vi "read_dust_control_settings_big.vi"(7 "Settings to be loaded":i32=-1, 8 "error in (no error)":errorcluster, 9 "Query Cluster":T1, 10 "Lower Timestamp Range":timestamp, 11 "Upper Timestamp Range":timestamp) -> (0 "error out":errorcluster, 1 "Settings Array":cluster{"String":string, "Value":dbl}[](array[cluster]), 3 "Dust Source Array":T2[](array[typedef]) {"Needle Voltage" min=0.0 max=10.0 step=0.01 format="%.2g"; "Y Voltage" min=0.0 max=9.0 step=0.01 format="%.2g"; "X Voltage" min=0.0 max=9.0 step=0.01 format="%.2g"; "Einzel Voltage" min=0.0 max=10.0 step=0.01 format="%.2g"; "Desired Amplitude (V)" min=0.0 max=10.0 step=0.01 format="%5.2f"; "Width (ms) : 0.1" min=0.05 max=5.0 step=0.01 format="%6.2f"; "Frequency" min=1.0 max=100.0 step=0.01 format="%.1f"})   [LabVIEW 2013]
doc: "Returns an array of events from the source_settings table based on the tag, dust type, high voltage, and id_source_settings, if specified. Unless a specific id_source_settings is requested, an uppper timestamp range and lower timestamp range are necessary."
uses:
  User Interface/Controls/dust_source_control.ctl
  <vilib>/addons/database/_DB Variant To Data/Database Variant To Data.xnode
panel:
  out "SQL Query Syntax":string
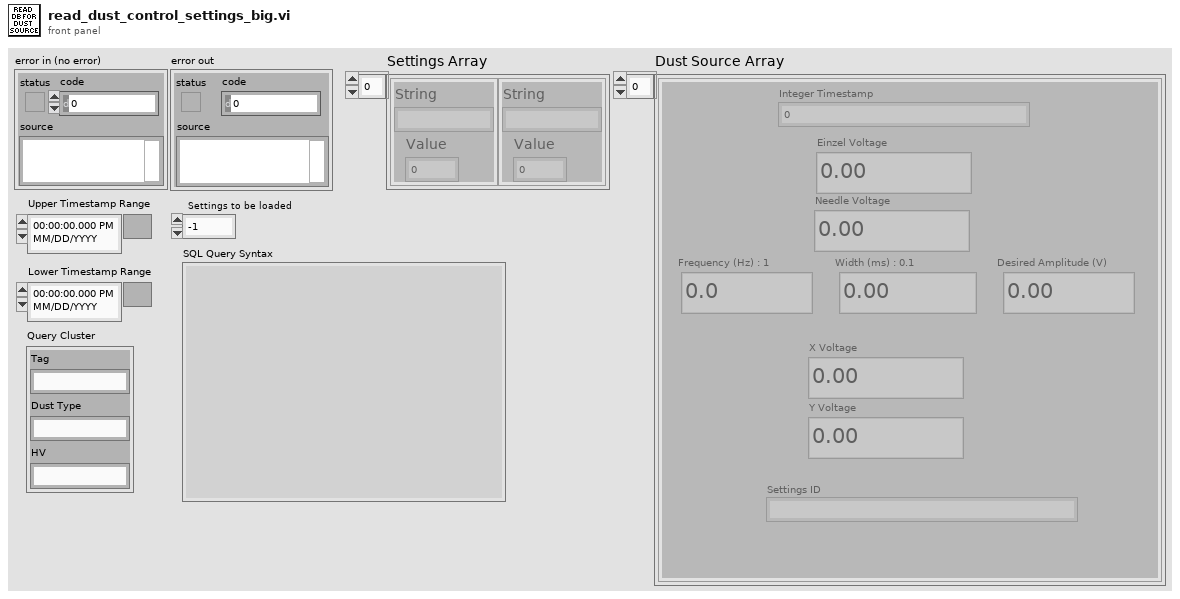
[diagram p1: front panel]
types:
  T1 = cluster{"Tag":string, "Dust Type":string, "HV":string}
  T2 = typedef "dust_source_control.ctl" = cluster{"Integer Timestamp":u64, "Einzel Voltage":dbl, "Needle Voltage":dbl, "Frequency":dbl, "Width (ms) : 0.1 ":dbl, "Desired Amplitude (V)":dbl, "X Voltage":dbl, "Y Voltage":dbl, "Settings ID":string, "ID#":i32}
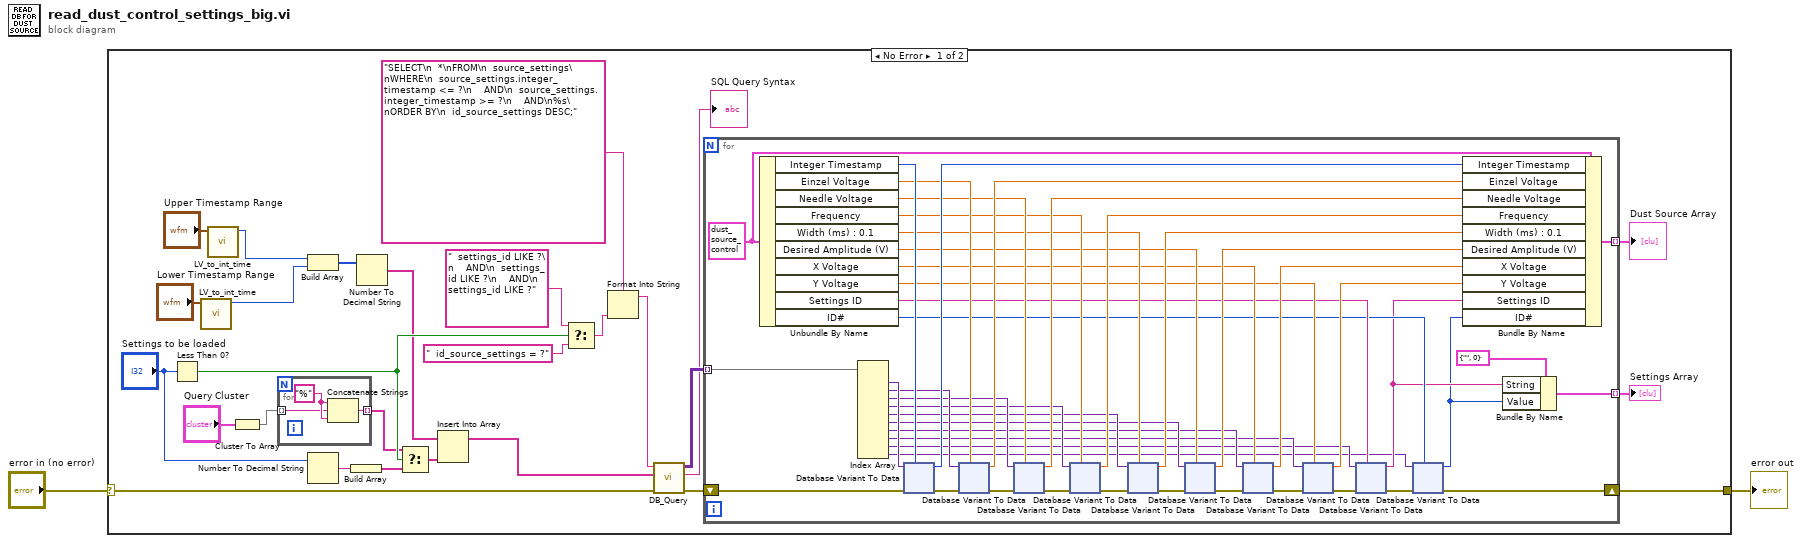
[diagram p0: block diagram]
diagram:
  n1 = case shown="No Error" "error in (no error)" {
    selector: "error in (no error)" -> [w9 w399]
    tunnel: [w24 w399] -> w1
    frame No Error {
      n2 = Less Than 0?(x="Settings to be loaded") -> (x < 0?=w19:bool)
      n3 = call "LV_to_int_time.vi"("Time Stamp"="Lower Timestamp Range") -> ("Integer Time"=w20:i64)  [unwired: 8 in, 1 out]
      n4 = call "LV_to_int_time.vi"("Time Stamp"="Upper Timestamp Range") -> ("Integer Time"=w21:i64)  [unwired: 8 in, 1 out]
      n5 = Cluster To Array(cluster="Query Cluster") -> (array=w7:string[])
      n6 = for {
        tunnel: w7 -> [w31] mode=indexing
        tunnel: [w30] -> w6 mode=indexing
        w32 = "%" ("string")
        n7 = Concatenate Strings(w32, w31, w32) -> (w30:string)
      }
      n8 = Build Array(w21, w20) -> (w18:i64[])
      n9 = Number To Decimal String(number="Settings to be loaded") -> (decimal integer string=w15:string)  [unwired: 1 in]
      n10 = Build Array(w15) -> (w14:string[])
      n11 = Number To Decimal String(number=w18) -> (decimal integer string=w13:string[])  [unwired: 1 in]
      n12 = Select(t=w6, s=w19, f=w14) -> (s? t:f=w12:string[])
      n13 = Insert Into Array(array=w13, new element=w12) -> (w10:string[])  [unwired: 1 in]
      n14 = Select(t="  settings_id LIKE ?\n    AND\n  settings_id LIKE ?\n    AND\n  settings_id LIKE ?" ("string"), s=w19, f="  id_source_settings = ?" ("string")) -> (s? t:f=w4:string)
      n15 = Format Into String(format string="SELECT\n  *\nFROM\n  source_settings\nWHERE\n  source_settings.integer_timestamp <= ?\n    AND\n  source_settings.integer_timestamp >= ?\n    AND\n%s\nORDER BY\n  id_source_settings DESC;" ("string"), w4) -> (resulting string=w3:string)  [unwired: 2 in, 1 out]
      n16 = call "DB_Query.vi"("error in (no error)"=w9, "Parameters"=w10, "Parameterized Query"=w3) -> ("error out"=w25:errorcluster, "Query in Standard Format"=→"SQL Query Syntax":string, "Results"=w26:variant[][])  [unwired: 6 in]
      n17 = for {
        tunnel: w26 -> [w59] mode=indexing
        shift-right: [w39] -> w24
        shift-left: w25 -> [w78]
        tunnel: [w62] -> w27 mode=indexing
        tunnel: [w36] -> w8 mode=indexing
        w60 = T2 {"Integer Timestamp"=0, "Einzel Voltage"=0.0, "Needle Voltage"=0.0, "Frequency"=1.0, "Width (ms) : 0.1 "=0.05, "Desired Amplitude (V)"=0.0, "X Voltage"=0.0, "Y Voltage"=0.0, "Settings ID"="", "ID#"=0} ("Dust Source Controls")
        n18 = Unbundle By Name(w60) -> ("Integer Timestamp"=w58:u64, "Einzel Voltage"=w56:dbl, "Needle Voltage"=w54:dbl, "Frequency"=w52:dbl, "Width (ms) : 0.1"=w50:dbl, "Desired Amplitude (V)"=w47:dbl, "X Voltage"=w45:dbl, "Y Voltage"=w44:dbl, "Settings ID"=w42:string, "ID#"=w38:i32)
        n19 = Index Array(array=w59) -> (element #1=w57:variant, element #2=w55:variant, element #3=w53:variant, element #4=w51:variant, element #5=w49:variant, element #6=w48:variant, element #7=w46:variant, element #8=w43:variant, element #9=w41:variant, element #10=w33:variant)  [unwired: 10 in]
        n20 = xnode "Database Variant To Data"("database variant"=w57, "error in"=w78, "type"=w58) -> ("data"=w61:u64, "error out"=w76:errorcluster)
        n21 = xnode "Database Variant To Data"("database variant"=w55, "error in"=w76, "type"=w56) -> ("data"=w77:dbl, "error out"=w74:errorcluster)
        n22 = xnode "Database Variant To Data"("database variant"=w53, "error in"=w74, "type"=w54) -> ("data"=w75:dbl, "error out"=w72:errorcluster)
        n23 = xnode "Database Variant To Data"("database variant"=w51, "error in"=w72, "type"=w52) -> ("data"=w73:dbl, "error out"=w70:errorcluster)
        n24 = xnode "Database Variant To Data"("database variant"=w49, "error in"=w70, "type"=w50) -> ("data"=w71:dbl, "error out"=w69:errorcluster)
        n25 = xnode "Database Variant To Data"("database variant"=w48, "error in"=w69, "type"=w47) -> ("data"=w68:dbl, "error out"=w66:errorcluster)
        n26 = xnode "Database Variant To Data"("database variant"=w46, "error in"=w66, "type"=w45) -> ("data"=w67:dbl, "error out"=w64:errorcluster)
        n27 = xnode "Database Variant To Data"("database variant"=w43, "error in"=w64, "type"=w44) -> ("data"=w65:dbl, "error out"=w63:errorcluster)
        n28 = xnode "Database Variant To Data"("database variant"=w41, "error in"=w63, "type"=w42) -> ("data"=w35:string, "error out"=w40:errorcluster)
        n29 = xnode "Database Variant To Data"("database variant"=w33, "error in (no error)"=w40, "type"=w38) -> ("data"=w34:i32, "error out"=w39:errorcluster)
        n30 = Bundle By Name(cluster=w60, "Integer Timestamp"=w61, "Einzel Voltage"=w77, "Needle Voltage"=w75, "Frequency"=w73, "Width (ms) : 0.1"=w71, "Desired Amplitude (V)"=w68, "X Voltage"=w67, "Y Voltage"=w65, "Settings ID"=w35, "ID#"=w34) -> (w62:T2)
        n31 = Bundle By Name(cluster=cluster{"String":string, "Value":i32} {"String"="", "Value"=0}, "String"=w35, "Value"=w34) -> (w36:cluster{"String":string, "Value":i32})
      }
      "Dust Source Array" <- w27
      "Settings Array" <- w8
    }
    frame Error {
    }
  }
  "error out" <- w1
